vi "BRig_dataRT_stats__init.vi"() -> (3 "output_dataRT_stats":u16[](array[numeric]))   [LabVIEW 2014]
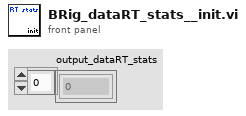
[diagram p1: front panel]
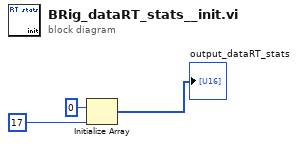
[diagram p0: block diagram]
diagram:
  n1 = Initialize Array(u16 0 ("element"), 17 ("dimension size")) -> (→"output_dataRT_stats":u16[])
